vi "Do.vi"(8 "error in":errorcluster, 10 "Actor in":refnum<class "Actor.lvclass">, 11 "Change File Writing State MSG":refnum<class "Change File Writing State MSG.lvclass">) -> (0 "error out":errorcluster, 2 "Actor out":refnum<class "Actor.lvclass">)   [LabVIEW 2017, in "File Library.lvlib" / "Change File Writing State MSG.lvclass"]
doc: "(<B>Filename</B>: Actor Framework.lvlib:Message.lvclass:Do.vi)\n\nDefines what a message does when it is received by an actor. Generally, a message instructs an actor to invoke one of its methods. By default, this method does nothing. A child class must override it to define behavior. Create a child class by using the Actor Framework Message Maker dialog box."
uses:
  Change File Writing State MSG.lvclass
  <vilib>/ActorFramework/Actor/Actor.lvclass
  File Actor.lvclass
  C:/Program Files (x86)/National Instruments/LabVIEW 2017/vi.lib/ActorFramework/Actor/Actor.lvclass
  File Actor.lvclass/File Actor.ctl
  Change File Writing State MSG.lvclass/Change File Writing State MSG.ctl
  Read Save DVR.vi
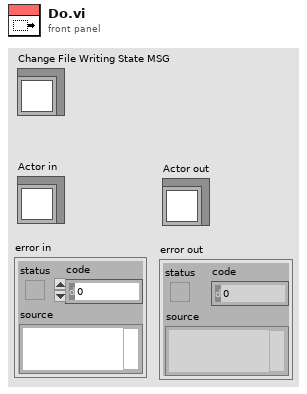
[diagram p1: front panel]
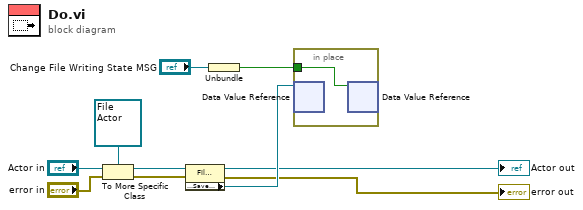
[diagram p0: block diagram]
diagram:
  n1 = To More Specific Class(target class=refnum<class "File Actor.lvclass"> refnum ("File Library.lvlib:File Actor"), reference="Actor in", error in="error in") -> (specific class reference=w6:refnum<class "File Actor.lvclass">, error out=w1:errorcluster)
  n2 = property class="File Actor"(reference=w6, error in=w1) -> (reference out=→"Actor out":refnum<class "File Actor.lvclass">, error out=→"error out":errorcluster, "Accessors:Save DVR"=w5:refnum<data-value>)
  n3 = Unbundle("Change File Writing State MSG") -> (w4:bool)
  n4 = in-place {
    in-place-border: w4 -> [w11]
    n5 = in-place-dvr #1(w5) -> ()  [unwired: 2 out]
    n6 = in-place-dvr #1(w11) -> ()  [unwired: 2 out]
  }
